vi "Impedance tube v0.9.vi"() -> ()   [LabVIEW 2021]
uses:
  <vilib>/Analysis/1siggen.llb/Ramp Pattern by Samples.vi
  <vilib>/express/express analysis/Spectral/Block/exnSpectralBlock spectral measurements RMS poly.vi
  <vilib>/express/express analysis/Spectral/Block/exnSpectralBlock spectral measurements RMS DDT.vi
  <vilib>/express/express arith-compare/Formula/XNode/ExpressFormulaBlockNode.xnode
  <vilib>/express/express analysis/Spectral/XNode/ExpressSpectralMeasurementsBlockNode.xnode
  <vilib>/Analysis/NI_AALPro.lvlib
  <vilib>/Analysis/NI_AALBase.lvlib
panel:
  out "Probe":dbl[](graph)
  out "Rr":dbl[](graph)
  out "Absorption coeff":dbl[](graph)
  in  "number of samples":i32=2048
  out "MIC 2":dynamicdata(graph)
  out "MIC 2":dbl
  out "FFT1":dynamicdata(graph)
  out "MIC 1":dynamicdata(graph)
  out "MIC 1":dbl
  in  "stop (F)":bool
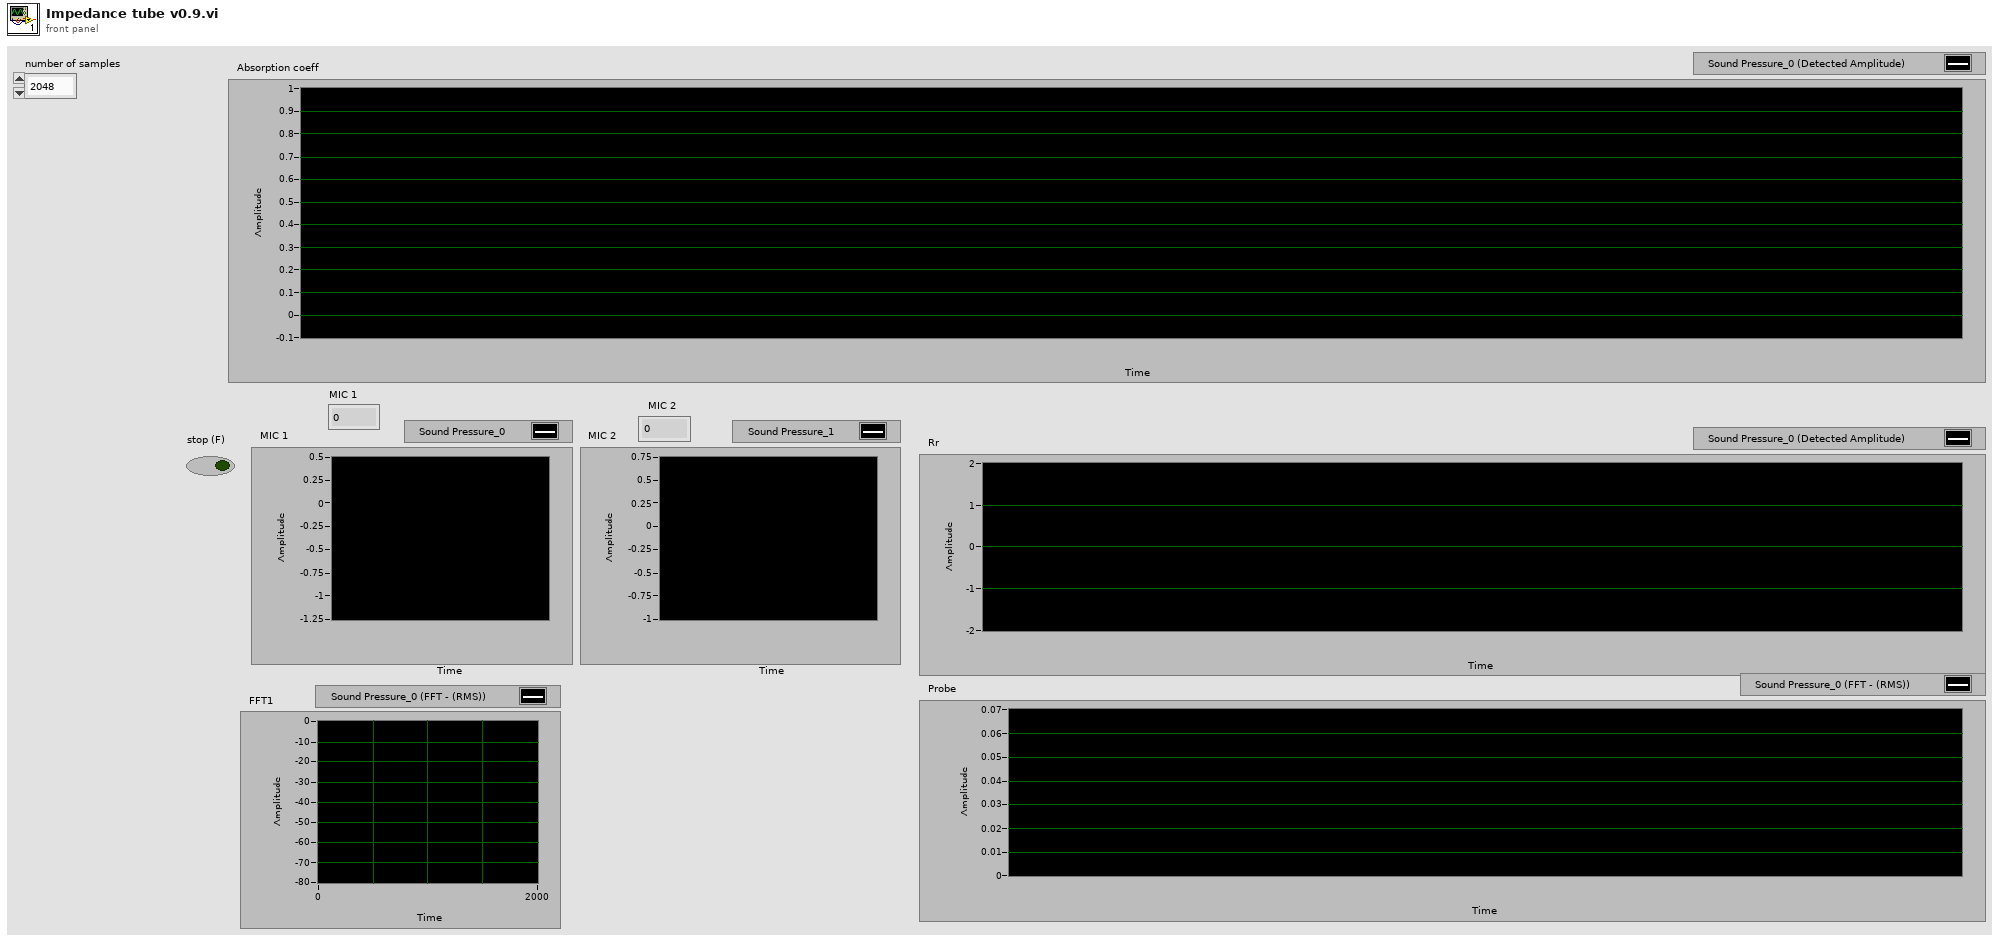
[diagram p1: front panel]
types:
  T1 = cluster{"averaging mode":u16, "weighting mode":u16, "number of averages":u32}
  T2 = cluster{"dB On (F)":bool, "unwrap phase (F)":bool, "convert to degree (F)":bool}
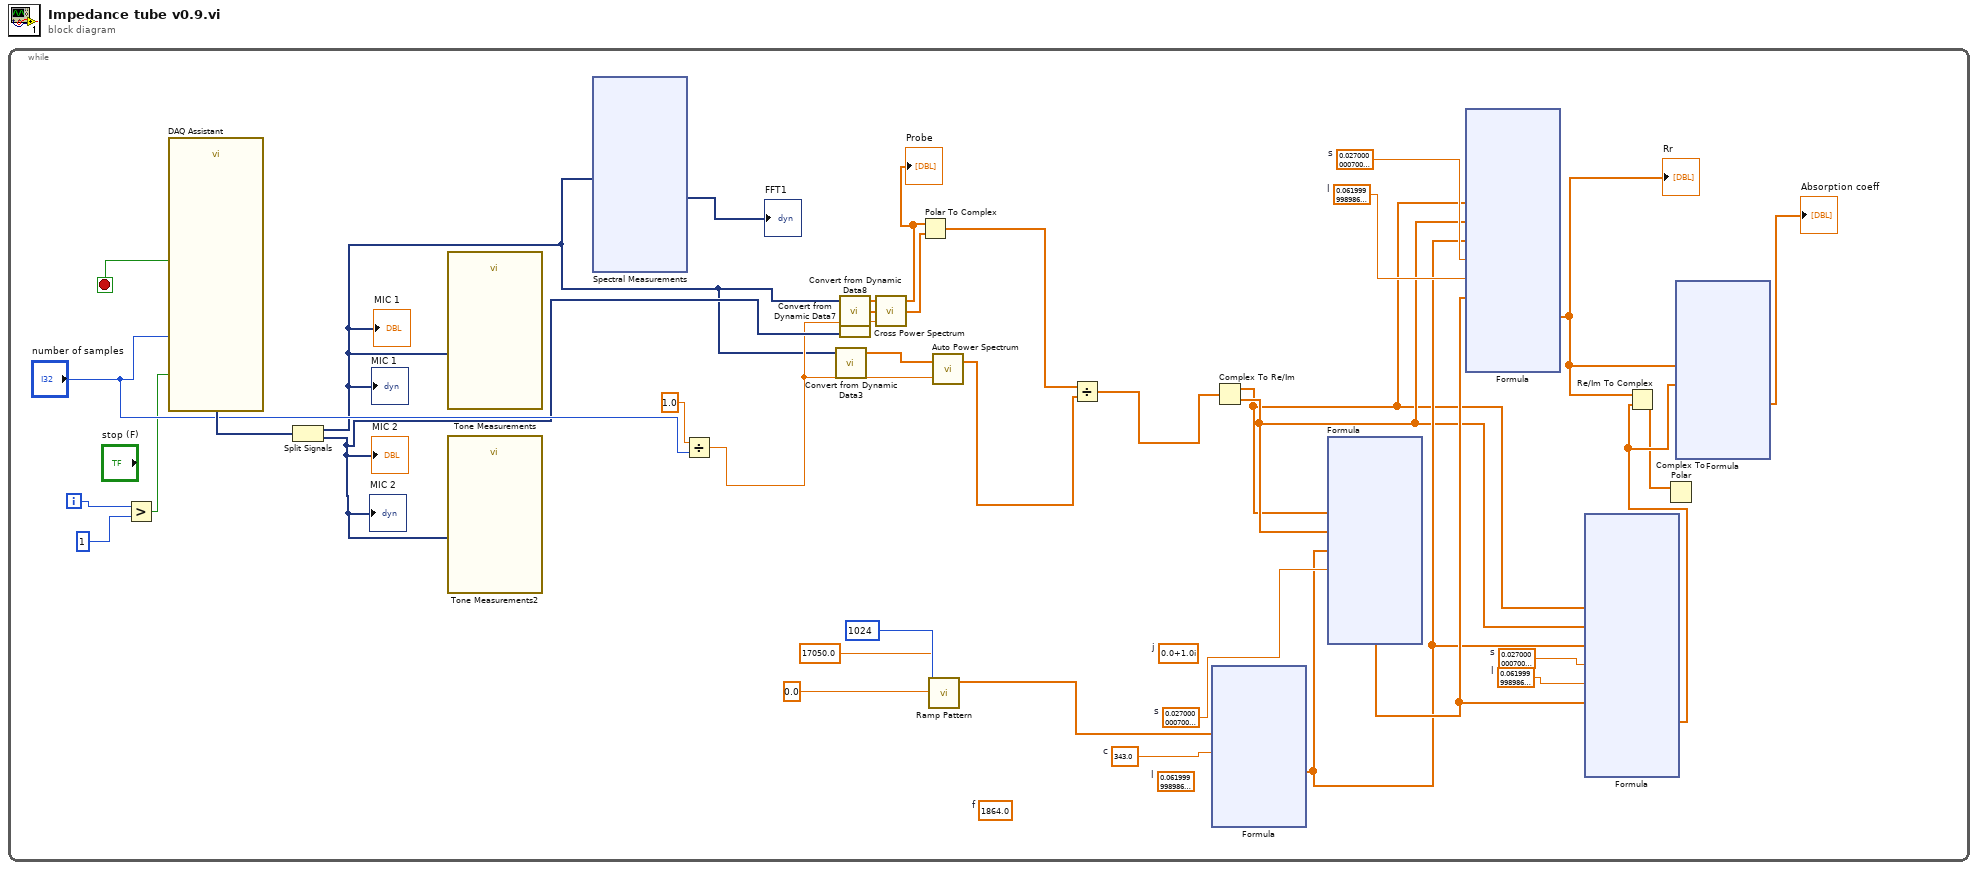
[diagram p0: block diagram]
diagram:
  n1 = while {
    i -> [w25]
    stop <- w37 stop-if-true
    w30 = sgl 0.062  # l
    w31 = sgl 0.027  # s
    w32 = sgl 0.062  # l
    w33 = sgl 0.027  # s
    (unwired) sgl 0.062  # l
    (unwired) sgl 1864.0  # f
    w34 = sgl 0.027  # s
    w35 = sgl 343.0  # c
    (unwired) csg 0.0+1.0i  # j
    n2 = Greater?(x=w25, y=1) -> (0:w18:bool)
    n3 = call "DAQ Assistant"("number of samples"="number of samples", "stop (F)"=w18) -> ("data"=w36:dynamicdata, "stopped"=w37:bool)  [unwired: 14 in, 2 out]
    n4 = Split Signals(w36) -> (w10:dynamicdata, w15:dynamicdata)  [unwired: 2 in]
    "MIC 1" <- w10
    "MIC 1" <- w10
    "MIC 2" <- w15
    "MIC 2" <- w15
    n5 = call "Tone Measurements"("Signals"=w10) -> ()  [unwired: 8 in, 3 out]
    n6 = call "Tone Measurements2"("Signals"=w15) -> ()  [unwired: 8 in, 3 out]
    n7 = xnode "Spectral Measurements"("Signals"=w10) -> ("FFT - (RMS)"=→"FFT1":dynamicdata)  [unwired: 1 in, 2 out]
    n8 = Divide(x=1.0, y="number of samples") -> (x/y=w12:dbl)
    n9 = call "Convert from Dynamic Data3"("Dynamic Data Type"=w10) -> ("Array"=w9:dbl[])  [unwired: 3 in]
    n10 = call "Convert from Dynamic Data7"("Dynamic Data Type"=w10) -> ("Array"=w16:dbl[])  [unwired: 3 in]
    n11 = call "Convert from Dynamic Data8"("Dynamic Data Type"=w15) -> ("Array"=w14:dbl[])  [unwired: 3 in]
    n12 = call <vilib>:"Cross Power Spectrum.vi"("dt"=w12, "Signal Y (V)"=w14, "Signal X (V)"=w16) -> ("Cross Power XY Spectrum Phase (radians)"=w13:dbl[], "Cross Power XY Spectrum Mag (V^2rms)"=w11:dbl[])  [unwired: 1 out]
    "Probe" <- w11
    n13 = Polar To Complex(1:w13, 2:w11) -> (0:w8:cdb[])
    n14 = call-poly <vilib>:"Ramp Pattern.vi"("start"=0.0, "end"=17050.0, "samples"=1024) -> ("Ramp Pattern"=w1:dbl[])  [unwired: 7 in, 1 out]
    n15 = call <vilib>:"Auto Power Spectrum.vi"("dt"=w12, "Signal (V)"=w9) -> ("Power Spectrum (V^2 rms)"=w7:dbl[])  [unwired: 1 out]
    n16 = Divide(x=w8, y=w7) -> (x/y=w6:cdb[])
    n17 = xnode "Formula"("f"=w1, "c"=w35) -> ("Result"=w28:dbl[])  [unwired: 1 in, 1 out]
    n18 = Complex To Re/Im(x + iy=w6) -> (x=w22:dbl[], y=w27:dbl[])
    n19 = xnode "Formula"("Hr"=w22, "Hi"=w27, "k"=w28, "s"=w34) -> ("Result"=w29:dbl[])  [unwired: 1 in, 1 out]
    n20 = xnode "Formula"("Hr"=w22, "Hi"=w27, "k"=w28, "s"=w33, "l"=w32, "D"=w29) -> ("Result"=w19:dbl[])  [unwired: 1 in, 1 out]
    "Rr" <- w19
    n21 = xnode "Formula"("Hr"=w22, "Hi"=w27, "k"=w28, "s"=w31, "l"=w30, "D"=w29) -> ("Result"=w26:dbl[])  [unwired: 1 in, 1 out]
    n22 = Re/Im To Complex(1:w26, 2:w19) -> (0:w23:cdb[])
    n23 = Complex To Polar(r * e^(i*theta)=w23) -> ()  [unwired: 2 out]
    n24 = xnode "Formula"("Rr"=w19, "Ri"=w26) -> ("Result"=→"Absorption coeff":dbl[])  [unwired: 1 in, 1 out]
  }
